vi "Print Polymorphic VI Instances.vi"(6 "Images Destination":path=path "", 8 "Error In":errorcluster, 11 "InstanceVIs":T1(array[cluster])) -> (0 "Error Out":errorcluster)   [LabVIEW 2018, in "Scripts.lvlib"]
uses:
  Scripts.lvlib
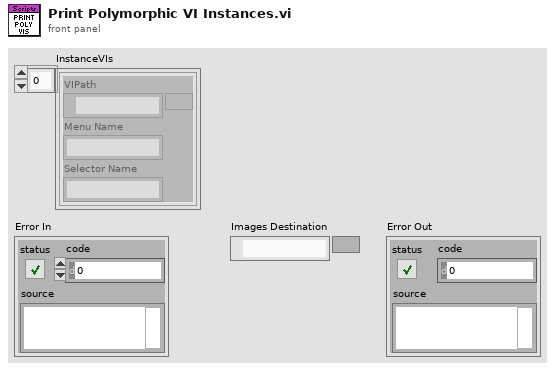
[diagram p1: front panel]
types:
  T1 = cluster{"VIPath":path, "Menu Name":string, "Selector Name":string}[]
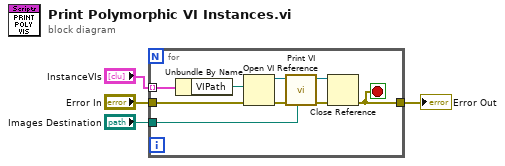
[diagram p0: block diagram]
diagram:
  n1 = for {
    tunnel: "InstanceVIs" -> [w13] mode=indexing
    tunnel: "Error In" -> [w11]
    tunnel: "Images Destination" -> [w5]
    tunnel: [w6] -> w4
    stop <- w6 stop-if-true
    n2 = Unbundle By Name(w13) -> ("VIPath"=w12:path)
    n3 = Open VI Reference(vi path=w12, error in (no error)=w11) -> (vi reference=w10:refnum<vi>, error out=w9:errorcluster)  [unwired: 4 in]
    n4 = call "Print VI.vi"("Images Destination"=w5, "Error In"=w9, "VI In"=w10) -> ("Error Out"=w7:errorcluster, "VI Out"=w8:refnum<vi>)  [unwired: 7 in]
    n5 = Close Reference(reference=w8, error in (no error)=w7) -> (error out=w6:errorcluster)
  }
  "Error Out" <- w4
